vi "HOL_TRAJECTORY_EXECUTE_SWERVE.vi"(4 "Time Offset":dbl=-1.0 format="%16.4f", 6 "EnableClosedLoop":bool=TRUE, 8 "Init":bool, 9 "Reverse":bool, 10 "Follow Orientation":bool, 11 "Gyro Heading\nRAD":dbl) -> (0 "AtReference":bool, 1 "OutputTRAJ_STATE":T6={"TimeSeconds"=0.0, "Velocity"=0.0, "Acceleration"=0.0, "POSE"={"TRANSLATION"={"X"=0.0, "Y"=0.0}, "ROTATION"={"VALUE"=0.0, "COS"=1.0, "SIN"=0.0}}, "Curvature"=0.0} {"POSE"."ROTATION"."SIN" format="%13.4f"; "POSE"."ROTATION"."COS" format="%13.4f"; "POSE"."ROTATION"."VALUE" format="%13.4f"; "POSE"."TRANSLATION"."Y" format="%14.3f"; "POSE"."TRANSLATION"."X" format="%14.3f"}, 2 "Error and Corr":T4 {"Error Pose"."ROTATION"."SIN" format="%13.4f"; "Error Pose"."ROTATION"."COS" format="%13.4f"; "Error Pose"."ROTATION"."VALUE" format="%13.4f"; "Error Pose"."TRANSLATION"."Y" format="%14.3f"; "Error Pose"."TRANSLATION"."X" format="%14.3f"}, 3 "Chassis Velocity Target":T5 {"vOmega" format="%10.3f"; "vY" format="%10.3f"; "vX" format="%10.3f"}, 5 "Orientation Target":dbl)   [LabVIEW 2019]
uses:
  <vilib>/Rock Robotics/WPI/ThirdParty/JAS_Junk/TrajLib/TypeDef/TRAJ_STATE.ctl
  <vilib>/Rock Robotics/WPI/ThirdParty/JAS_Junk/TrajLib/TypeDef/POSE2D.ctl
  <vilib>/Rock Robotics/WPI/ThirdParty/JAS_Junk/TrajLib/TypeDef/TRANSLATION2D.ctl
  <vilib>/Rock Robotics/WPI/ThirdParty/JAS_Junk/TrajLib/TypeDef/ROTATION2D.ctl
  <vilib>/Rock Robotics/WPI/ThirdParty/JAS_Junk/TrajLib/TypeDef/CHASSIS_SPEEDS.ctl
  <vilib>/Rock Robotics/WPI/ThirdParty/JAS_Junk/TrajLib/ProfiledPIDController_NewPeriod.vi
  <vilib>/Rock Robotics/WPI/ThirdParty/JAS_Junk/TrajLib/ProfiledPIDController_SetIntegratorRange.vi
  <vilib>/Rock Robotics/WPI/ThirdParty/JAS_Junk/TrajLib/ProfiledPIDController_DisableContInput.vi
  <vilib>/Rock Robotics/WPI/ThirdParty/JAS_Junk/TrajLib/ProfiledPIDController_EnableContInput.vi
  <vilib>/Rock Robotics/WPI/ThirdParty/JAS_Junk/TrajLib/TrapProfConstraint_New.vi
  <vilib>/Rock Robotics/WPI/ThirdParty/JAS_Junk/TrajLib/MathUtil_InputModulus.vi
  <vilib>/Rock Robotics/WPI/ThirdParty/JAS_Junk/TrajLib/Translation2d_Create.vi
  <vilib>/Rock Robotics/WPI/ThirdParty/JAS_Junk/TrajLib/HolDrvCtrl_New.vi
  <vilib>/Rock Robotics/WPI/ThirdParty/JAS_Junk/TrajLib/HolDrvCtrl_PackPID.vi
  <vilib>/Rock Robotics/WPI/ThirdParty/JAS_Junk/TrajLib/HolDrvCtrl_SetTolerance.vi
  <vilib>/Rock Robotics/WPI/ThirdParty/JAS_Junk/TrajLib/HolDrvCtrl_SetEnabled.vi
  <vilib>/Rock Robotics/WPI/ThirdParty/JAS_Junk/TrajLib/HolDrvCtrl_Calculate_Trajectory.vi
  <vilib>/Rock Robotics/WPI/ThirdParty/JAS_Junk/TrajLib/HolDrvCtrl_AtReference.vi
  <vilib>/Rock Robotics/WPI/ThirdParty/JAS_Junk/TrajLib/Rotation2d_UnaryMinus.vi
  <vilib>/Rock Robotics/WPI/ThirdParty/JAS_Junk/TrajLib/Rotation2d_RotateBy.vi
  <vilib>/Rock Robotics/WPI/ThirdParty/JAS_Junk/TrajLib/TrapProfState_New.vi
  <vilib>/Rock Robotics/WPI/ThirdParty/JAS_Junk/TrajLib/PIDController_NewPeriod.vi
  <vilib>/Rock Robotics/SystemInterfaces/NetworkCommunication/NetComm_UsageReport_report.vi
  <vilib>/Rock Robotics/WPI/ThirdParty/JAS_Junk/TrajLib/PIDController_SetIntegratorRange.vi
  <vilib>/Rock Robotics/WPI/ThirdParty/JAS_Junk/TrajLib/PIDController_DisableContinousInput.vi
  <vilib>/Rock Robotics/WPI/ThirdParty/JAS_Junk/TrajLib/PIDController_EnableContinousInput.vi
  <vilib>/Rock Robotics/WPI/ThirdParty/JAS_Junk/TrajLib/Conv_Deg_Radians.vi
  <vilib>/Rock Robotics/WPI/ThirdParty/JAS_Junk/TrajLib/PIDController_Reset.vi
  <vilib>/Rock Robotics/WPI/ThirdParty/JAS_Junk/TrajLib/HolDrvCtrl_Calculate.vi
  <vilib>/Rock Robotics/WPI/ThirdParty/JAS_Junk/TrajLib/Pose2d_getXYAngle.vi
  <vilib>/Rock Robotics/WPI/ThirdParty/JAS_Junk/TrajLib/Rotation2d_CreateXY.vi
  <vilib>/Rock Robotics/WPI/ThirdParty/JAS_Junk/TrajLib/ProfiledPIDController_Calculate_Meas_Goal.vi
  <vilib>/Rock Robotics/WPI/ThirdParty/JAS_Junk/TrajLib/ChassisSpeeds_FromFieldRelativeSpeeds.vi
  <vilib>/Rock Robotics/WPI/ThirdParty/JAS_Junk/TrajLib/PIDController_Calculate_SP_PV.vi
  <vilib>/Rock Robotics/WPI/ThirdParty/JAS_Junk/TrajLib/ProfiledPIDController_Reset_PosOnly.vi
  <vilib>/Rock Robotics/WPI/ThirdParty/JAS_Junk/TrajLib/Rotation2d_GetAngleCosSin.vi
  <vilib>/Rock Robotics/WPI/ThirdParty/JAS_Junk/TrajLib/Pose2d_RelativeTo.vi
  <vilib>/Rock Robotics/WPI/ThirdParty/JAS_Junk/TrajLib/Util_CalcDist.vi
  <vilib>/Rock Robotics/WPI/ThirdParty/JAS_Junk/TrajLib/ProfiledPIDController_SetGoal_PosOnly.vi
  <vilib>/Rock Robotics/WPI/ThirdParty/JAS_Junk/TrajLib/ProfiledPIDController_Calculate_Meas.vi
  <vilib>/Rock Robotics/WPI/ThirdParty/JAS_Junk/TrajLib/Rotation2d_GetCos.vi
  <vilib>/Rock Robotics/WPI/ThirdParty/JAS_Junk/TrajLib/Rotation2d_GetSin.vi
  <vilib>/Rock Robotics/WPI/ThirdParty/JAS_Junk/TrajLib/PIDController_SetSetpoint.vi
  <vilib>/Rock Robotics/WPI/ThirdParty/JAS_Junk/TrajLib/PIDController_Calculate_PV.vi
  <vilib>/Rock Robotics/WPI/ThirdParty/JAS_Junk/TrajLib/ProfiledPIDController_Reset.vi
  <vilib>/Rock Robotics/WPI/ThirdParty/JAS_Junk/TrajLib/Transform2d_Create_PosePose.vi
  <vilib>/Rock Robotics/WPI/ThirdParty/JAS_Junk/TrajLib/ProfiledPIDController_SetGoal.vi
  <vilib>/Rock Robotics/WPI/ThirdParty/JAS_Junk/TrajLib/TrapProfile_New.vi
  <vilib>/Rock Robotics/WPI/ThirdParty/JAS_Junk/TrajLib/ProfiledPIDController_GetPeriod.vi
  <vilib>/Rock Robotics/WPI/ThirdParty/JAS_Junk/TrajLib/TrapProfile_Calculate.vi
  <vilib>/Rock Robotics/WPI/ThirdParty/JAS_Junk/TrajLib/ControllerUtil_GetModulusError.vi
  <vilib>/Rock Robotics/WPI/ThirdParty/JAS_Junk/TrajLib/Translation2d_RotateBy.vi
  <vilib>/Rock Robotics/WPI/ThirdParty/JAS_Junk/TrajLib/Translation2d_Minus.vi
  <vilib>/Rock Robotics/WPI/ThirdParty/JAS_Junk/TrajLib/TrapProfile_ShouldFlipAcceleration.vi
  <vilib>/Rock Robotics/WPI/ThirdParty/JAS_Junk/TrajLib/TrapProfile_Direct.vi
  <vilib>/Rock Robotics/WPI/ThirdParty/JAS_Junk/TrajLib/PIDController_GetPeriod.vi
  <vilib>/Rock Robotics/WPI/ThirdParty/JAS_Junk/TrajLib/Util_LibraryGlobals.vi
  <vilib>/Rock Robotics/WPI/ThirdParty/JAS_Junk/TrajLib/Trajectory_Library.lvlib
panel:
  # "(FOR TESTING)"
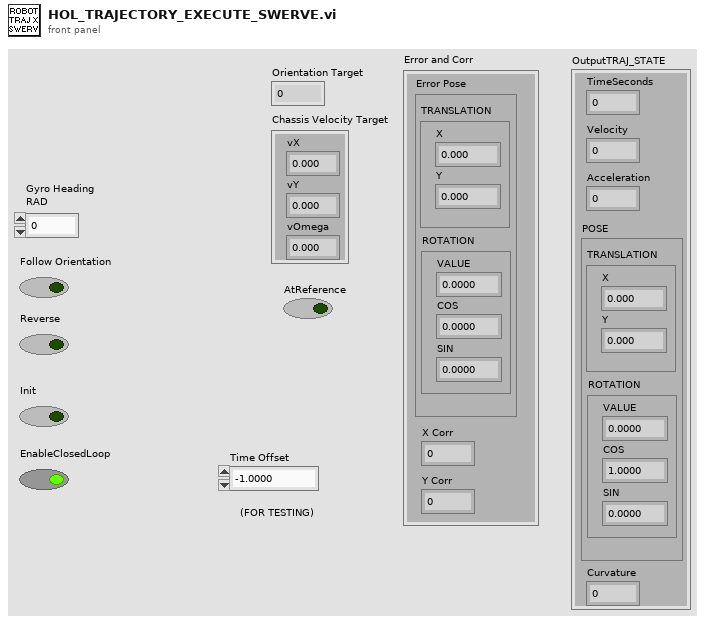
[diagram p1: front panel]
types:
  T1 = typedef "Trajectory_Library.lvlib/POSE2D.ctl" = cluster{"TRANSLATION":T2, "ROTATION":T3}
  T2 = typedef "Trajectory_Library.lvlib/TRANSLATION2D.ctl" = cluster{"X":dbl, "Y":dbl}
  T3 = typedef "Trajectory_Library.lvlib/ROTATION2D.ctl" = cluster{"VALUE":dbl, "COS":dbl, "SIN":dbl}
  T4 = cluster{"Error Pose":T1, "X Corr":dbl, "Y Corr":dbl}
  T5 = typedef "Trajectory_Library.lvlib/CHASSIS_SPEEDS.ctl" = cluster{"vX":dbl, "vY":dbl, "vOmega":dbl}
  T6 = typedef "Trajectory_Library.lvlib/TRAJ_STATE.ctl" = cluster{"TimeSeconds":dbl, "Velocity":dbl, "Acceleration":dbl, "POSE":T1, "Curvature":dbl}
  T7 = typedef "Trajectory_Library.lvlib/SWERVE_DRIVE_MODULE_POSITION.ctl" = cluster{"Distance":dbl, "Angle":T3, "P":bool}
  T8 = typedef "Trajectory_Library.lvlib/SWERVE_DRIVE_KINEMATICS.ctl" = cluster{"NumModules":i32, "InverseKinematics":T9, "ForwardKinematics":T9, "Modules":T2[], "PrevCoR":T2, "SavedModuleStates":T10[]}
  T9 = typedef "NI_Matrix.lvlib/RealMatrix.ctl" = dbl[][]
  T10 = typedef "Trajectory_Library.lvlib/SWERVE_DRIVE_MODULE_STATE.ctl" = cluster{"Speed":dbl, "Angle":T3}
  T11 = typedef "Trajectory_Library.lvlib/SWERVE_DRIVE_ODOMETRY.ctl" = cluster{"POSE":T1, "GyroOffset":T3, "PreviousAngle":T3, "PrevModulePositions":T7[], "NumModules":i32}
  T12 = typedef "Trajectory_Library.lvlib/TRAJECTORY.ctl" = cluster{"TotalTImeSecs":dbl, "States":T6[]}
  T13 = typedef "Trajectory_Library.lvlib/PID_TUNING.ctl" = cluster{"Kp":dbl, "Ki":dbl, "Kd":dbl, "MaximumIntegral":dbl, "MinimumIntegral":dbl}
  T14 = typedef "Trajectory_Library.lvlib/PROFILED_PID_CONTROLLER.ctl" = cluster{"Controller":T15, "Goal":T16, "Setpoint":T16, "Constraint":T17}
  T15 = typedef "Trajectory_Library.lvlib/PID_CONTROLLER.ctl" = cluster{"Kp":dbl, "Ki":dbl, "Kd":dbl, "Period":dbl, "Max_Integral":dbl, "Min_Integral":dbl, "Max_Input":dbl, "Min_Input":dbl, "Continuous":bool, "PositionError":dbl, "VelocityError":dbl, "PrevError":dbl, "TotalError":dbl, "PositionTolerance":dbl, "VelocityTolerance":dbl, "SetPoint":dbl, "Kf":dbl, "Prev_Deriv":dbl, "Prev_Deriv 2":dbl, "DerivativeFilter":bool, "Min_Output":dbl, "Max_Output":dbl, "Prev_F_P":dbl, "Prev_F_P_2":dbl, "AntiWindupActive":bool, "Measurement":dbl}
  T16 = typedef "Trajectory_Library.lvlib/TRAPEZOID_PROFILE_STATE.ctl" = cluster{"Position":dbl, "Velocity":dbl}
  T17 = typedef "Trajectory_Library.lvlib/TRAPEZOID_PROFILE_CONSTRAINT.ctl" = cluster{"MaxVelocity":dbl, "MaxAcceleration":dbl}
  T18 = typedef "Trajectory_Library.lvlib/HOLONOMIC_DRV_CTRL.ctl" = cluster{"poseTolerance":T1, "poseError":T1, "Enabled":bool, "PID_xCtrl":T15, "PID_yCtrl":T15, "PROF_PID_thetaCtrl":T14, "RotationError":T3, "FirstRun":bool}
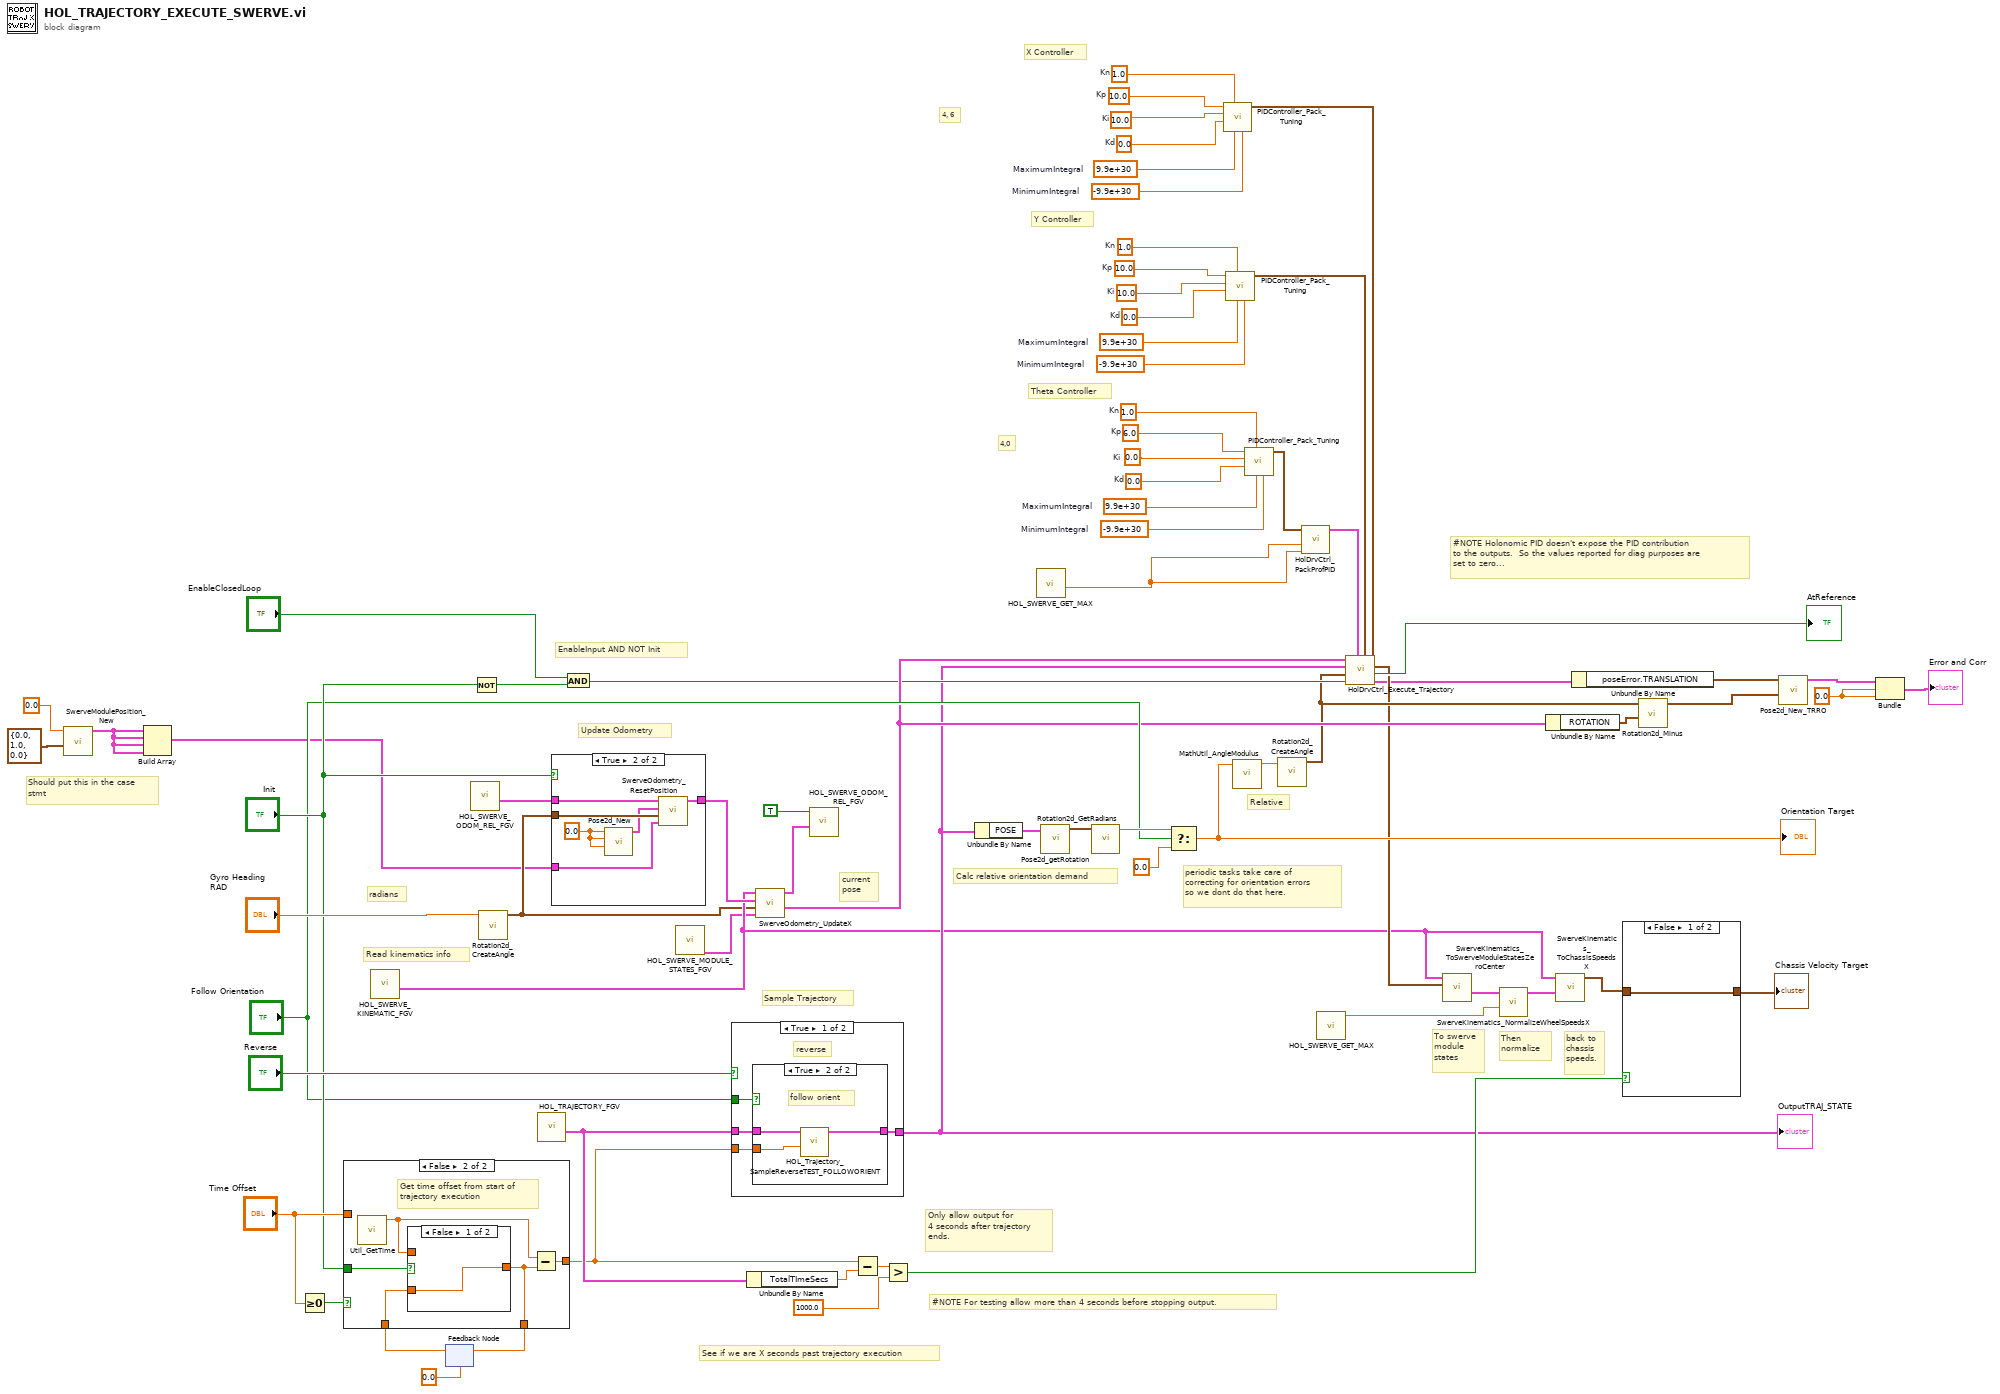
[diagram p0: block diagram]
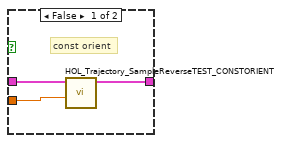
[diagram p4: hidden frame]
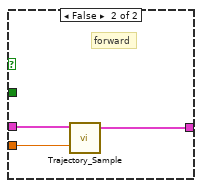
[diagram p5: hidden frame]
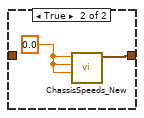
[diagram p7: hidden frame]
diagram:
  w24 = 1.0  # Kn
  w27 = 6.0  # Kp
  w36 = 0.0  # Ki
  w37 = 0.0  # Kd
  w38 = 9.9e+30  # MaximumIntegral
  w39 = -9.9e+30  # MinimumIntegral
  w22 = 1.0  # Kn
  w25 = 10.0  # Kp
  w28 = 10.0  # Ki
  w29 = 0.0  # Kd
  w30 = 9.9e+30  # MaximumIntegral
  w31 = -9.9e+30  # MinimumIntegral
  w23 = 1.0  # Kn
  w26 = 10.0  # Kp
  w32 = 10.0  # Ki
  w33 = 0.0  # Kd
  w34 = 9.9e+30  # MaximumIntegral
  w35 = -9.9e+30  # MinimumIntegral
  w51 = 0.0
  # "4,0"
  # "4, 6"
  # "Should put this in the case\nstmt"
  # "#NOTE For testing allow more than 4 seconds before stopping output."
  # "EnableInput AND NOT Init"
  # "Theta Controller"
  # "Y Controller"
  # "X Controller"
  # "Relative"
  # "#NOTE Holonomic PID doesn't expose the PID contribution \nto the outputs.  So the values reported for diag purposes are\nset to zero..."
  # "current\npose"
  # "back to\nchassis\nspeeds."
  # "Then\nnormalize"
  # "To swerve\nmodule\nstates"
  # "Calc relative orientation demand"
  # "Read kinematics info"
  # "Sample Trajectory"
  # "See if we are X seconds past trajectory execution"
  # "Update Odometry"
  # "radians"
  # "periodic tasks take care of\ncorrecting for orientation errors\nso we dont do that here."
  # "Only allow output for\n4 seconds after trajectory\nends."
  n1 = call <vilib>:"SwerveModulePosition_New.vi"("ROTATION"=T3 {"VALUE"=0.0, "COS"=1.0, "SIN"=0.0}, "Distance"=0.0) -> ("SWERVE_DRIVE_MODULE_POSITION"=w3:T7)  [unwired: 9 in]
  n2 = Build Array(w3, w3, w3, w3) -> (w2:T7[])
  n3 = Greater Or Equal To 0?(x="Time Offset") -> (x >= 0?=w55:bool)
  n4 = call "HOL_SWERVE_KINEMATIC_FGV.vi"() -> ("out SWERVE_DRIVE_KINEMATICS"=w8:T8)  [unwired: 11 in]
  n5 = feedback #1(0.0 ("TIME")) -> (w57:dbl)
  n6 = case shown="False" w55 {
    tunnel: [w76 w82] -> w73
    tunnel: "Init" -> [_ w80]
    tunnel: w57 -> [w77 w79]
    tunnel: [w77 w78] -> w56
    tunnel: "Time Offset" -> [w76 _]
    frame True {
      # "For testing allow\nuser entered time offset!!"
    }
    frame False {
      # "Get time offset from start of\ntrajectory execution"
      n7 = call <vilib>:"Util_GetTime.vi"() -> ("FPGA_Time_Seconds"=w81:dbl)  [unwired: 10 in, 1 out]
      n8 = case shown="False" w80 {
        tunnel: [w83 w84] -> w78
        tunnel: w79 -> [w83 _]
        tunnel: w81 -> [_ w84]
        frame False {
        }
        frame True {
        }
      }
      n9 = Subtract(x=w81, y=w78) -> (x-y=w82:dbl)
    }
  }
  n10 = feedback-in #1(w56) -> ()
  n11 = call "HOL_SWERVE_ODOM_REL_FGV.vi"() -> ("out SWERVE_DRIVE_ODOMETRY"=w68:T11)  [unwired: 11 in]
  n12 = Not(x="Init") -> (.not. x?=w52:bool)
  n13 = call <vilib>:"Rotation2d_CreateAngle.vi"("Angle"="Gyro Heading\nRAD") -> ("ROTATION"=w7:T3)  [unwired: 10 in]
  n14 = call "HOL_TRAJECTORY_FGV.vi"() -> ("outTRAJECTORY"=w75:T12)  [unwired: 11 in]
  n15 = case shown="True" "Init" {
    tunnel: w68 -> [w85 w91]
    tunnel: [w85 w90] -> w9
    tunnel: w7 -> [_ w89]
    tunnel: w2 -> [_ w86]
    frame False {
    }
    frame True {
      w88 = 0.0 ("X")
      n16 = call <vilib>:"Pose2d_New.vi"("Heading"=w88, "Y"=w88, "X"=w88) -> ("out POSe"=w87:T1)  [unwired: 8 in]
      n17 = call <vilib>:"SwerveOdometry_ResetPosition.vi"("Module Positions"=w86, "gyroAngle"=w89, "Pose"=w87, "in SWERVE_DRIVE_ODOMETRY"=w91) -> ("out SWERVE_DRIVE_ODOMETRY"=w90:T11)  [unwired: 6 in, 1 out]
    }
  }
  n18 = And(x="EnableClosedLoop", y=w52) -> (x .and. y?=w15:bool)
  n19 = call "HOL_SWERVE_MODULE_STATES_FGV.vi"() -> ("Out Current Module Positions"=w6:T7[])  [unwired: 10 in, 1 out]
  n20 = case shown="True" "Reverse" {
    tunnel: w75 -> [w95 w104]
    tunnel: w73 -> [w93 w103]
    tunnel: [w94 w102] -> w14
    tunnel: "Follow Orientation" -> [w92 _]
    frame True {
      # "reverse"
      n21 = case shown="True" w92 {
        tunnel: w95 -> [w98 w101]
        tunnel: [w96 w100] -> w94
        tunnel: w93 -> [w97 w99]
        frame False {
          # "const orient"
          n22 = call "HOL_Trajectory_SampleReverseTEST_CONSTORIENT.vi"("Time"=w97, "InputTRAJECTORY"=w98) -> ("OutputTRAJ_STATE"=w96:T6)  [unwired: 9 in]
        }
        frame True {
          # "follow orient"
          n23 = call "HOL_Trajectory_SampleReverseTEST_FOLLOWORIENT.vi"("Time"=w99, "InputTRAJECTORY"=w101) -> ("OutputTRAJ_STATE"=w100:T6)  [unwired: 9 in]
        }
      }
    }
    frame False {
      # "forward"
      n24 = call <vilib>:"Trajectory_Sample.vi"("Time"=w103, "InputTRAJECTORY"=w104) -> ("OutputTRAJ_STATE"=w102:T6)  [unwired: 9 in]
    }
  }
  "OutputTRAJ_STATE" <- w14
  n25 = Unbundle By Name(w75) -> ("TotalTImeSecs"=w74:dbl)
  n26 = call <vilib>:"SwerveOdometry_UpdateX.vi"("module Positions"=w6, "gyroAngle"=w7, "in SWERVE_DRIVE_ODOMETRY"=w9, "SWERVE_DRIVE_KINEMATICS"=w8) -> ("robot POSE"=w16:T1, "out SWERVE_DRIVE_ODOMETRY"=w62:T11)  [unwired: 5 in, 1 out]
  n27 = call "HOL_SWERVE_ODOM_REL_FGV.vi"("in SWERVE_DRIVE_ODOMETRY"=w62, "WRITE"=TRUE) -> ()  [unwired: 9 in, 1 out]
  n28 = Subtract(x=w73, y=w74) -> (x-y=w72:dbl)
  n29 = Greater?(x=w72, y=1000.0) -> (0:w70:bool)
  n30 = Unbundle By Name(w14) -> ("POSE"=w59:T1)
  n31 = call "HOL_SWERVE_GET_MAX.vi"() -> ("Max Rotational Vel (Rad/Sec)"=w17:dbl)  [unwired: 10 in, 1 out]
  n32 = call <vilib>:"Pose2d_getRotation.vi"("in POSE"=w59) -> ("out ROTATION"=w64:T3)  [unwired: 10 in]
  n33 = call <vilib>:"Rotation2d_GetRadians.vi"("in ROTATION"=w64) -> ("AngleRadians"=w43:dbl)  [unwired: 10 in]
  n34 = Select(t=w43, s="Follow Orientation", f=0.0) -> (s? t:f=w40:dbl)
  "Orientation Target" <- w40
  n35 = call <vilib>:"PIDController_Pack_Tuning.vi"("MinimumIntegral"=w31, "MaximumIntegral"=w30, "Kn"=w22, "Kd"=w29, "Ki"=w28, "Kp"=w25) -> ("PID Tuning"=w18:T13)  [unwired: 5 in]
  n36 = call <vilib>:"PIDController_Pack_Tuning.vi"("MinimumIntegral"=w35, "MaximumIntegral"=w34, "Kn"=w23, "Kd"=w33, "Ki"=w32, "Kp"=w26) -> ("PID Tuning"=w19:T13)  [unwired: 5 in]
  n37 = call <vilib>:"MathUtil_AngleModulus.vi"("InputAngle"=w40) -> ("ModulsAngle"=w49:dbl)  [unwired: 10 in]
  n38 = call <vilib>:"PIDController_Pack_Tuning.vi"("MinimumIntegral"=w39, "MaximumIntegral"=w38, "Kn"=w24, "Kd"=w37, "Ki"=w36, "Kp"=w27) -> ("PID Tuning"=w21:T13)  [unwired: 5 in]
  n39 = call <vilib>:"Rotation2d_CreateAngle.vi"("Angle"=w49) -> ("ROTATION"=w13:T3)  [unwired: 10 in]
  n40 = call <vilib>:"HolDrvCtrl_PackProfPID.vi"("Max Accel"=w17, "Max Speed"=w17, "Theta PID Tuning"=w21) -> ("Theta PID CONTROLLER"=w20:T14)  [unwired: 8 in]
  n41 = call "HOL_SWERVE_GET_MAX.vi"() -> ("Max Wheel Vel (Meter/Sec)"=w60:dbl)  [unwired: 10 in, 1 out]
  n42 = call <vilib>:"HolDrvCtrl_Execute_Trajectory.vi"("X PID Tuning"=w18, "Y PID Tuning"=w19, "thetaProfiledPID_CTRL"=w20, "Enable"=w15, "angleRef"=w13, "desiredTrajState"=w14, "currentPose"=w16) -> ("outHOLONOMIC_DRV_CTRL"=w10:T18, "AtReference"=→"AtReference":bool, "calcChassisSpeed"=w11:T5)  [unwired: 2 in]
  n43 = call <vilib>:"SwerveKinematics_ToSwerveModuleStatesZeroCenter.vi"("ChassisSpeeds"=w11, "in SWERVE_DRIVE_KINEMATICS"=w8) -> ("ModuleStates"=w66:T10[])  [unwired: 8 in, 1 out]
  n44 = call <vilib>:"SwerveKinematics_NormalizeWheelSpeedsX.vi"("AttainableMaxSpeed"=w60, "in WheelStates"=w66) -> ("out WheelStates"=w65:T10[])  [unwired: 9 in]
  n45 = Unbundle By Name(w16) -> ("ROTATION"=w44:T3)
  n46 = call <vilib>:"SwerveKinematics_ToChassisSpeedsX.vi"("WheelStates"=w65, "in SWERVE_DRIVE_KINEMATICS"=w8) -> ("Chassis Speed"=w1:T5)  [unwired: 9 in]
  n47 = Unbundle By Name(w10) -> ("poseError.TRANSLATION"=w48:T2)
  n48 = case shown="False" w70 {
    tunnel: w1 -> [w105 _]
    tunnel: [w105 w106] -> w61
    frame False {
    }
    frame True {
      w107 = 0.0 ("vX")
      n49 = call <vilib>:"ChassisSpeeds_New.vi"("vAngular"=w107, "vY"=w107, "vX"=w107) -> ("CHASSIS"=w106:T5)  [unwired: 8 in]
    }
  }
  "Chassis Velocity Target" <- w61
  n50 = call <vilib>:"Rotation2d_Minus.vi"("other ROTATION"=w44, "in ROTATION"=w13) -> ("out ROTATION"=w47:T3)  [unwired: 9 in]
  n51 = call <vilib>:"Pose2d_New_TRRO.vi"("ROTATION"=w47, "TRANSLATION"=w48) -> ("outPOSE"=w46:T1)  [unwired: 9 in]
  n52 = Bundle("outPOSE"=w46, w51, w51) -> (→"Error and Corr":cluster{"outPOSE":T1, dbl, dbl})  [unwired: 1 in]
